vi "ROS_Topic_Write_Stop_Continuous_Primitive.vi"(3 "ROS in":T1) -> (1 "ROS out":T1)   [LabVIEW 2013]
doc: "Instructs the server to stop publishing messages continuously."
uses:
  SubVIs/_ROSControl.ctl
  SubVIs/_ROSDirection.ctl
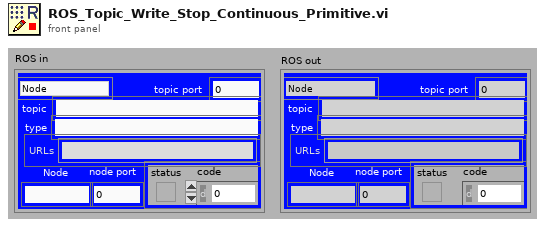
[diagram p1: front panel]
types:
  T1 = typedef "_ROSControl.ctl" = cluster{"topic port":u16, "Node":string, "topic":string, "type":string, "node port":u32, "error ":errorcluster, "Direction":T2, "APIs":string[]}
  T2 = typedef "_ROSDirection.ctl" = enum16{"Node", "Publisher", "Subscriber", "Service Client"}
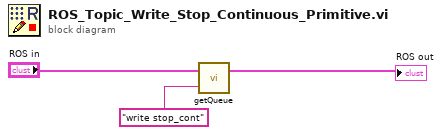
[diagram p0: block diagram]
diagram:
  n1 = call "getQueue.vi"("queue msg"="write stop_cont" ("t"), "ROS in"="ROS in") -> ("ROS out"=→"ROS out":T1)  [unwired: 1 in]
